vi "Status_toStatus.vi"(8 "error in (no error)":errorcluster, 9 "ms timeout (-1)":i32=-1, 10 "responseQ":string, 11 "Command":string) -> (0 "error out":errorcluster, 2 "response":string)   [LabVIEW 2016]
panel:
  in  "cmdstruct":cluster{"cmd":string, "respQ":string}
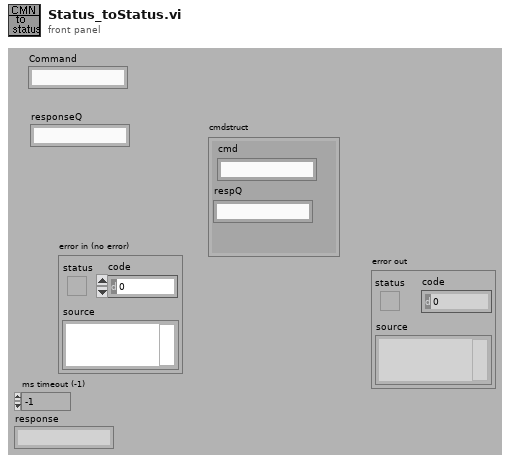
[diagram p1: front panel]
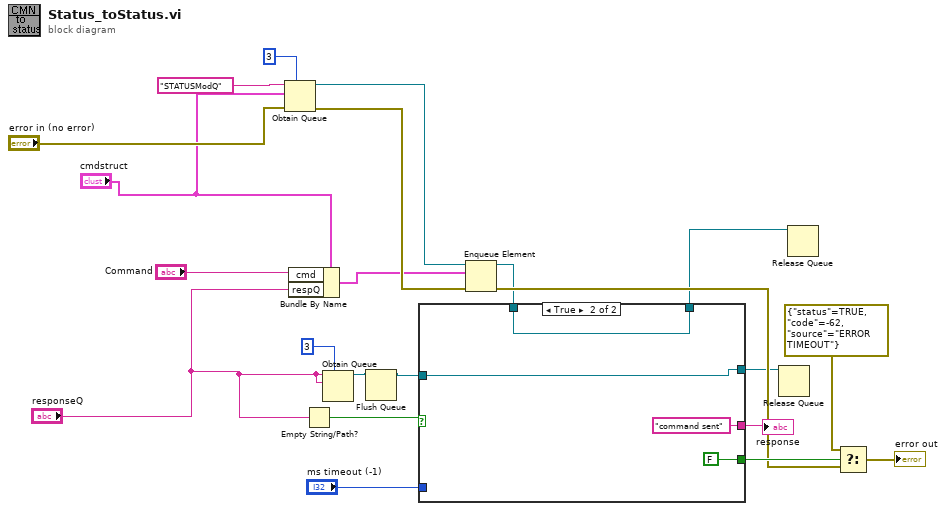
[diagram p0: block diagram]
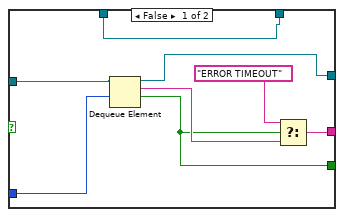
[diagram p2: hidden frame]
diagram:
  n1 = Obtain Queue(max queue size (-1, unlimited)=3, name (unnamed)="STATUSModQ", element data type="cmdstruct", error in (no error)="error in (no error)") -> (queue out=w21:refnum<queue>, error out=w15:errorcluster)  [unwired: 1 in, 1 out]
  n2 = Bundle By Name(cluster="cmdstruct", "cmd"="Command", "respQ"="responseQ") -> (w9:cluster{"cmd":string, "respQ":string})
  n3 = Empty String/Path?(string/path="responseQ") -> (empty?=w19:bool)
  n4 = Obtain Queue(max queue size (-1, unlimited)=3, name (unnamed)="responseQ", element data type="responseQ") -> (queue out=w6:refnum<queue>)  [unwired: 2 in, 2 out]
  n5 = Flush Queue(queue=w6) -> (queue out=w4:refnum<queue>)  [unwired: 1 in, 2 out]
  n6 = Enqueue Element(queue=w21, element=w9, error in (no error)=w15) -> (queue out=w7:refnum<queue>, error out=w11:errorcluster)  [unwired: 2 out]
  n7 = case shown="True" w19 {
    tunnel: "ms timeout (-1)" -> [w30 _]
    tunnel: [w27 "command sent"] -> w17
    tunnel: [w26 FALSE ("timed out?")] -> w14
    tunnel: [w25 w32] -> w8
    tunnel: w7 -> [w25 w32]
    tunnel: w4 -> [w24 w31]
    tunnel: [w23 w31] -> w3
    frame False {
      n8 = Dequeue Element(queue=w24, timeout in ms (-1)=w30) -> (queue out=w23:refnum<queue>, element=w29:string, timed out?=w26:bool)  [unwired: 1 in, 1 out]
      n9 = Select(t="ERROR TIMEOUT", s=w26, f=w29) -> (s? t:f=w27:string)
    }
    frame True {
    }
  }
  "response" <- w17
  n10 = Release Queue(queue=w3) -> ()  [unwired: 1 in, 4 out]
  n11 = Release Queue(queue=w8) -> ()  [unwired: 1 in, 4 out]
  n12 = Select(t=errorcluster {"status"=TRUE, "code"=-62, "source"="ERROR TIMEOUT"}, s=w14, f=w11) -> (s? t:f=→"error out":errorcluster)
